vi "Auto_Drive (2).vi"(11 "Drive Effort":dbl=-0.2) -> ()   [LabVIEW 2016]
uses:
  <vilib>/Rock Robotics/WPI/SafetyOutput/WPI_SafetyOutputConfigMenu.ctl
  Global 2.vi
panel:
  in  "Scaling Factor":dbl=-16.0 format="%#_13g"
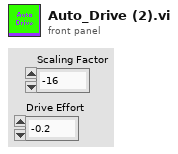
[diagram p1: front panel]
types:
  T1 = typedef "WPI_SafetyOutputConfigMenu.ctl" = enum16{"Enable", "Disable"}
  T2 = typedef "WPI_MotorControlDeviceRef.ctl" = cluster{"DeviceStatus":errorcluster, "Type":T3, "PWM":cluster{"PWM Channel":T4, "DeadBand":T5}, "CAN":cluster{"Device Number":u8, "SetOutput VI Ref":variant, "GetOutput VI Ref":variant, "Enable VI Ref":variant, "Disable VI Ref":variant, "Data":variant}, "Invert":bool}
  T3 = typedef "WPI_MotorControlType.ctl" = enum16{"PWM", "CAN"}
  T4 = typedef "FPGA_DIOPWMChannel.ctl" = enum8{"PWM 0", "PWM 1", "PWM 2", "PWM 3", "PWM 4", "PWM 5", "PWM 6", "PWM 7", "PWM 8", "PWM 9", "PWM MXP 0", "PWM MXP 1", "PWM MXP 2", "PWM MXP 3", "PWM MXP 4", "PWM MXP 5", "PWM MXP 6", "PWM MXP 7", "PWM MXP 8", "PWM MXP 9", "Invalid"}
  T5 = typedef "WPI_PWMDeadband.ctl" = cluster{"Name":string, "maxPositivePwm":i32, "minPositivePwm":i32, "centerPwm":i32, "maxNegativePwm":i32, "minNegativePwm":i32, "angularRange":u16}
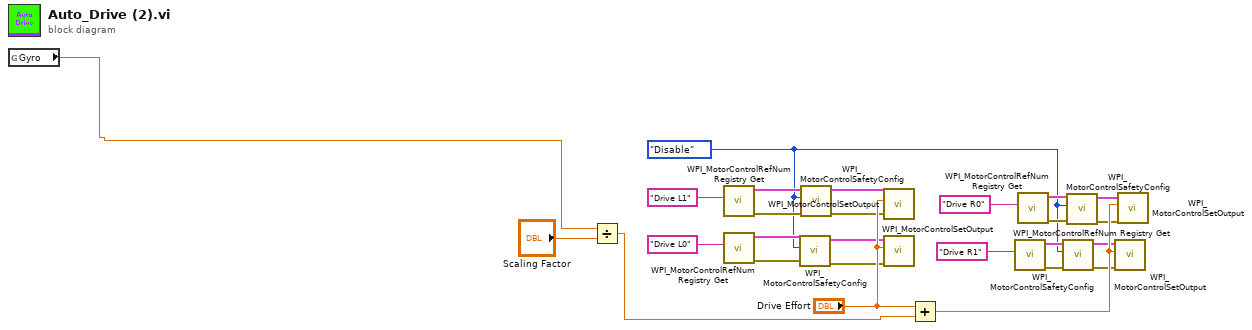
[diagram p0: block diagram]
diagram:
  w4 = WPI_SafetyOutputConfigMenu."Disable" ("mode")
  n1 = global read "Global 2.vi" "Gyro"() -> (w1:dbl)
  n2 = Divide(x=w1, y="Scaling Factor") -> (x/y=w2:dbl)
  n3 = call <vilib>:"WPI_MotorControlRefNum Registry Get.vi"("refnum name"="Drive L1") -> ("error out"=w19:errorcluster, "MotorControlDevRef"=w20:T2)  [unwired: 9 in]
  n4 = call <vilib>:"WPI_MotorControlRefNum Registry Get.vi"("refnum name"="Drive L0") -> ("error out"=w15:errorcluster, "MotorControlDevRef"=w16:T2)  [unwired: 9 in]
  n5 = call <vilib>:"WPI_MotorControlSafetyConfig.vi"("error in (no error)"=w15, "mode"=w4, "MotorControlDevRef"=w16) -> ("error out"=w13:errorcluster, "MotorControlDevRef"=w14:T2)  [unwired: 7 in]
  n6 = call <vilib>:"WPI_MotorControlSafetyConfig.vi"("error in (no error)"=w19, "mode"=w4, "MotorControlDevRef"=w20) -> ("error out"=w17:errorcluster, "MotorControlDevRef"=w18:T2)  [unwired: 7 in]
  n7 = call <vilib>:"WPI_MotorControlSetOutput.vi"("error in (no error)"=w17, "Output"="Drive Effort", "MotorControlDevRef"=w18) -> ()  [unwired: 6 in, 3 out]
  n8 = call <vilib>:"WPI_MotorControlSetOutput.vi"("error in (no error)"=w13, "Output"="Drive Effort", "MotorControlDevRef"=w14) -> ()  [unwired: 6 in, 3 out]
  n9 = Add(x="Drive Effort", y=w2) -> (x+y=w22:dbl)
  n10 = call <vilib>:"WPI_MotorControlRefNum Registry Get.vi"("refnum name"="Drive R1") -> ("error out"=w7:errorcluster, "MotorControlDevRef"=w8:T2)  [unwired: 9 in]
  n11 = call <vilib>:"WPI_MotorControlRefNum Registry Get.vi"("refnum name"="Drive R0") -> ("error out"=w11:errorcluster, "MotorControlDevRef"=w12:T2)  [unwired: 9 in]
  n12 = call <vilib>:"WPI_MotorControlSafetyConfig.vi"("error in (no error)"=w7, "mode"=w4, "MotorControlDevRef"=w8) -> ("error out"=w6:errorcluster, "MotorControlDevRef"=w5:T2)  [unwired: 7 in]
  n13 = call <vilib>:"WPI_MotorControlSafetyConfig.vi"("error in (no error)"=w11, "mode"=w4, "MotorControlDevRef"=w12) -> ("error out"=w10:errorcluster, "MotorControlDevRef"=w9:T2)  [unwired: 7 in]
  n14 = call <vilib>:"WPI_MotorControlSetOutput.vi"("error in (no error)"=w6, "Output"=w22, "MotorControlDevRef"=w5) -> ()  [unwired: 6 in, 3 out]
  n15 = call <vilib>:"WPI_MotorControlSetOutput.vi"("error in (no error)"=w10, "Output"=w22, "MotorControlDevRef"=w9) -> ()  [unwired: 6 in, 3 out]
